vi "Selected items for S4P Tool.vi"(10 "Item Syms":i32[](array[numeric]), 11 "Item name":string[](array[string])) -> (1 "Selected tem index":i32[](array[numeric]), 2 "Item Seleced?":bool, 3 "Selected tem":string[](array[string]))   [LabVIEW 2011]
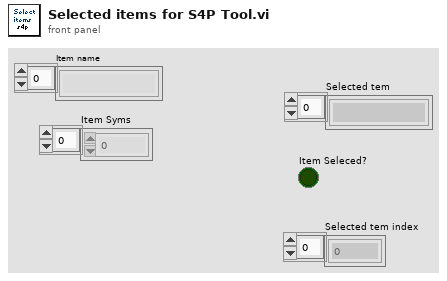
[diagram p1: front panel]
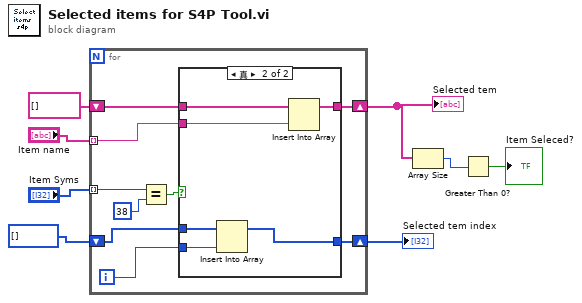
[diagram p0: block diagram]
diagram:
  n1 = for {
    tunnel: "Item name" -> [w13] mode=indexing
    tunnel: "Item Syms" -> [w17] mode=indexing
    shift-right: [w12] -> w5
    shift-left: string[] [] ("Item name") -> [w14]
    shift-right: [w9] -> w1
    shift-left: i32[] [] ("Item Syms") -> [w11]
    i -> [w10]
    n2 = Equal?(x=w17, y=38) -> (x = y?=w15:bool)
    n3 = case shown="真" w15 {
      tunnel: w14 -> [w19 w25]
      tunnel: w13 -> [_ w20]
      tunnel: [w19 w22] -> w12
      tunnel: w11 -> [w18 w24]
      tunnel: w10 -> [_ w21]
      tunnel: [w18 w23] -> w9
      frame False {
      }
      frame True {
        n4 = Insert Into Array(array=w24, new element=w21) -> (w23:i32[])  [unwired: 1 in]
        n5 = Insert Into Array(array=w25, new element=w20) -> (w22:string[])  [unwired: 1 in]
      }
    }
  }
  "Selected tem" <- w5
  "Selected tem index" <- w1
  n6 = Array Size(array=w5) -> (size(s)=w3:i32)
  n7 = Greater Than 0?(x=w3) -> (x > 0?=→"Item Seleced?":bool)
